vi "FPGA_DMA_Init_5160.vi"(8 "error in (no error)":errorcluster, 11 "FPGA VI Reference":T1) -> (0 "error out":errorcluster, 3 "FPGA VI Reference out":T1, 5 "Remaining":u32)   [LabVIEW 2013]
uses:
  Config/5160FPGAref.ctl
  <vilib>/rvi/interface/common/niFpgaWaitOnOcc.vi
  <vilib>/Utility/error.llb/Error Cluster From Error Code.vi
  <vilib>/rvi/errors/niLvFpgaAdjustHostInterfaceError.vi
  <vilib>/rvi/interface/nirviMethod/nirviMethod.xnode
  <vilib>/rvi/errors/niLvFpgaMergeErrorWithErrorCode.vi
  <vilib>/FPGAPlugInAG/Dynamic/niLvFpga_ReadFifo_Dynamic.vi
  <vilib>/FPGAPlugInAG/Dynamic/niLvFpga_ConfigureFifo_Dynamic.vi
  <vilib>/FPGAPlugInAG/Dynamic/niLvFpga_StartFifo_Dynamic.vi
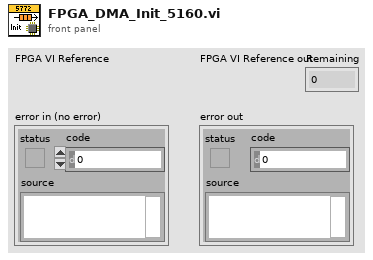
[diagram p1: front panel]
types:
  T1 = typedef "5160FPGAref.ctl" = refnum<k20>
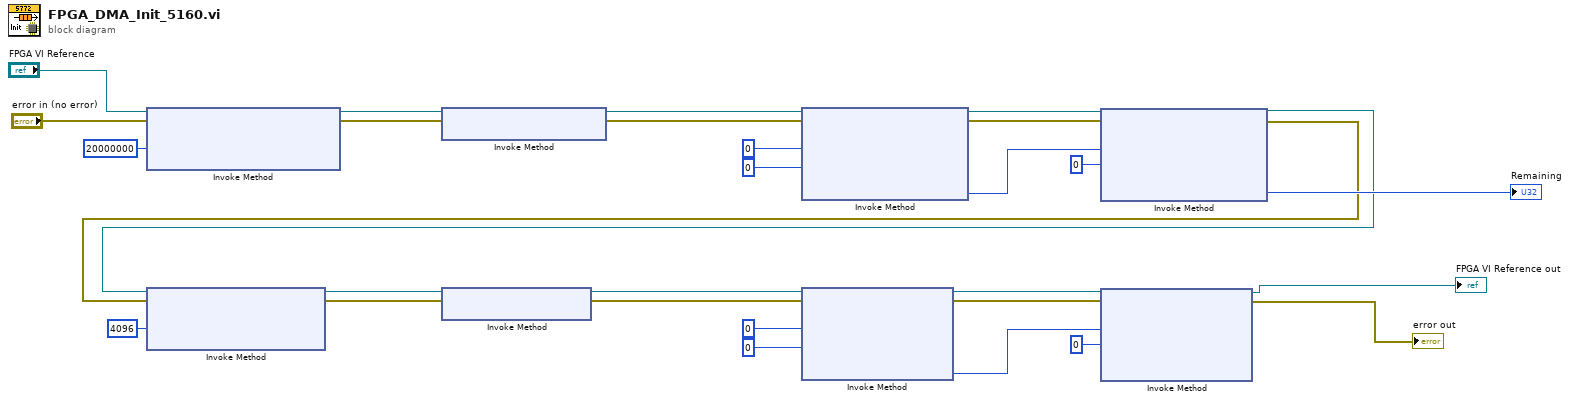
[diagram p0: block diagram]
diagram:
  n1 = xnode "Invoke Method"("FPGA VI Reference In"="FPGA VI Reference", "error in"="error in (no error)", "Requested Depth"=u32 20000000 ("Depth")) -> ("FPGA VI Reference Out"=w25:T1, "error out"=w26:errorcluster)  [unwired: 1 out]
  n2 = xnode "Invoke Method"("FPGA VI Reference In"=w25, "error in"=w26) -> ("FPGA VI Reference Out"=w16:T1, "error out"=w18:errorcluster)
  n3 = xnode "Invoke Method"("FPGA VI Reference In"=w16, "error in"=w18, "Number of Elements"=u32 0, "Timeout (ms)"=0) -> ("FPGA VI Reference Out"=w20:T1, "error out"=w19:errorcluster, "Elements Remaining"=w22:u32)  [unwired: 1 out]
  n4 = xnode "Invoke Method"("FPGA VI Reference In"=w20, "error in"=w19, "Number of Elements"=w22, "Timeout (ms)"=0) -> ("FPGA VI Reference Out"=w4:T1, "error out"=w1:errorcluster, "Elements Remaining"=→"Remaining":u32)  [unwired: 1 out]
  n5 = xnode "Invoke Method"("FPGA VI Reference In"=w4, "error in"=w1, "Requested Depth"=u32 4096 ("Depth")) -> ("FPGA VI Reference Out"=w7:T1, "error out"=w6:errorcluster)  [unwired: 1 out]
  n6 = xnode "Invoke Method"("FPGA VI Reference In"=w7, "error in"=w6) -> ("FPGA VI Reference Out"=w15:T1, "error out"=w14:errorcluster)
  n7 = xnode "Invoke Method"("FPGA VI Reference In"=w15, "error in"=w14, "Number of Elements"=u32 0, "Timeout (ms)"=0) -> ("FPGA VI Reference Out"=w12:T1, "error out"=w13:errorcluster, "Elements Remaining"=w10:u32)  [unwired: 1 out]
  n8 = xnode "Invoke Method"("FPGA VI Reference In"=w12, "error in"=w13, "Number of Elements"=w10, "Timeout (ms)"=0) -> ("FPGA VI Reference Out"=→"FPGA VI Reference out":T1, "error out"=→"error out":errorcluster)  [unwired: 2 out]
